vi "play_nPoint_id_slew_OL_FIFO.vi"() -> ()   [LabVIEW 2017]
uses:
  <vilib>/Analysis/Matrix/Datatypes/RealMatrix.ctl
  <vilib>/userdefined/High Color/nirio_resource_hc.ctl
  <vilib>/FPGAPlugInAG/cRIO-9082/niLvFpga_Open_cRIO-9082.vi
  <vilib>/rvi/interface/common/dynamic/niFpgaDynamicAddResources.vi
  <vilib>/FPGAPlugInAG/Dynamic/niLvFpga_Reset_Dynamic.vi
  <vilib>/rvi/interface/common/niFpgaWaitOnOcc.vi
  <vilib>/Utility/error.llb/Error Cluster From Error Code.vi
  <vilib>/rvi/errors/niLvFpgaAdjustHostInterfaceError.vi
  <vilib>/Analysis/Matrix/Numeric/Conversions/Matrix To Array - RM.vi
  <vilib>/FPGAPlugInAG/Dynamic/niLvFpga_Run_Dynamic.vi
  <vilib>/Analysis/Matrix/Numeric/Conversions/Array To Matrix - RA2.vi
  <vilib>/FPGAPlugInAG/Dynamic/niLvFpga_Close_Dynamic.vi
  <vilib>/rvi/interface/nirviOpenFPGA/nirviOpenFPGA.xnode
  FPGA Bitfiles/afmimagingcontro_FPGATargetSPARTA_IDOLFIFOinput_8nsqzYocPkw.lvbitx
  <vilib>/rvi/interface/nirviMethod/nirviMethod.xnode
  <vilib>/rvi/interface/nirviReadWriteControl/nirviReadWriteControl.xnode
  <vilib>/rvi/interface/nirviCloseFPGA/nirviCloseFPGA.xnode
  <vilib>/rvi/errors/niLvFpgaMergeErrorWithErrorCode.vi
  <vilib>/FPGAPlugInAG/Dynamic/niLvFpga_ConfigureFifo_Dynamic.vi
  <vilib>/rvi/interface/Simulation/niFpgaSimulationCallBeginRW.vi
  <vilib>/FPGAPlugInAG/Dynamic/niLvFpga_WriteFifo_Dynamic.vi
  <vilib>/FPGAPlugInAG/Dynamic/niLvFpga_ReadFifo_Dynamic.vi
  NiFpgaLv.dll
  <vilib>/Utility/file.llb/Read Delimited Spreadsheet (DBL).vi
  <vilib>/Analysis/Matrix/NI_Matrix.lvlib
  <vilib>/Utility/file.llb/Write Delimited Spreadsheet (DBL).vi
panel:
  out "stage_data_out":T1
  in  "u_in":T1
  in  "DAC-select":i16
  out "Timed Out?":bool
  out "Waveform Graph":dbl[](graph)
  out "Actual Depth 2":u32
  out "unsigned 16bit integer":u16
  out "Elements Remaining":u32
  out "Actual Depth":u32
  out "error out":errorcluster
  out "size(s) 3":i32[](array[numeric])
  out "x+y":i32
  out "YK TO":bool
  out "Unstable Traj":bool
  in  "traj_in_path":path
  out "AI1":T2(graph)
  out "size(s) 2":i32[](array[numeric])
  in  "data_out_path":path
  out "AI0":T2(graph)
  out "Waveform Chart":T2(graph)
  out "Loop Done":bool
  in  "Abort":bool
  in  "TsTicks":u32=1600
  out "y iter":i32
  out "size(s)":i32
  in  "umax":dbl=4.0 format="%#_13g"
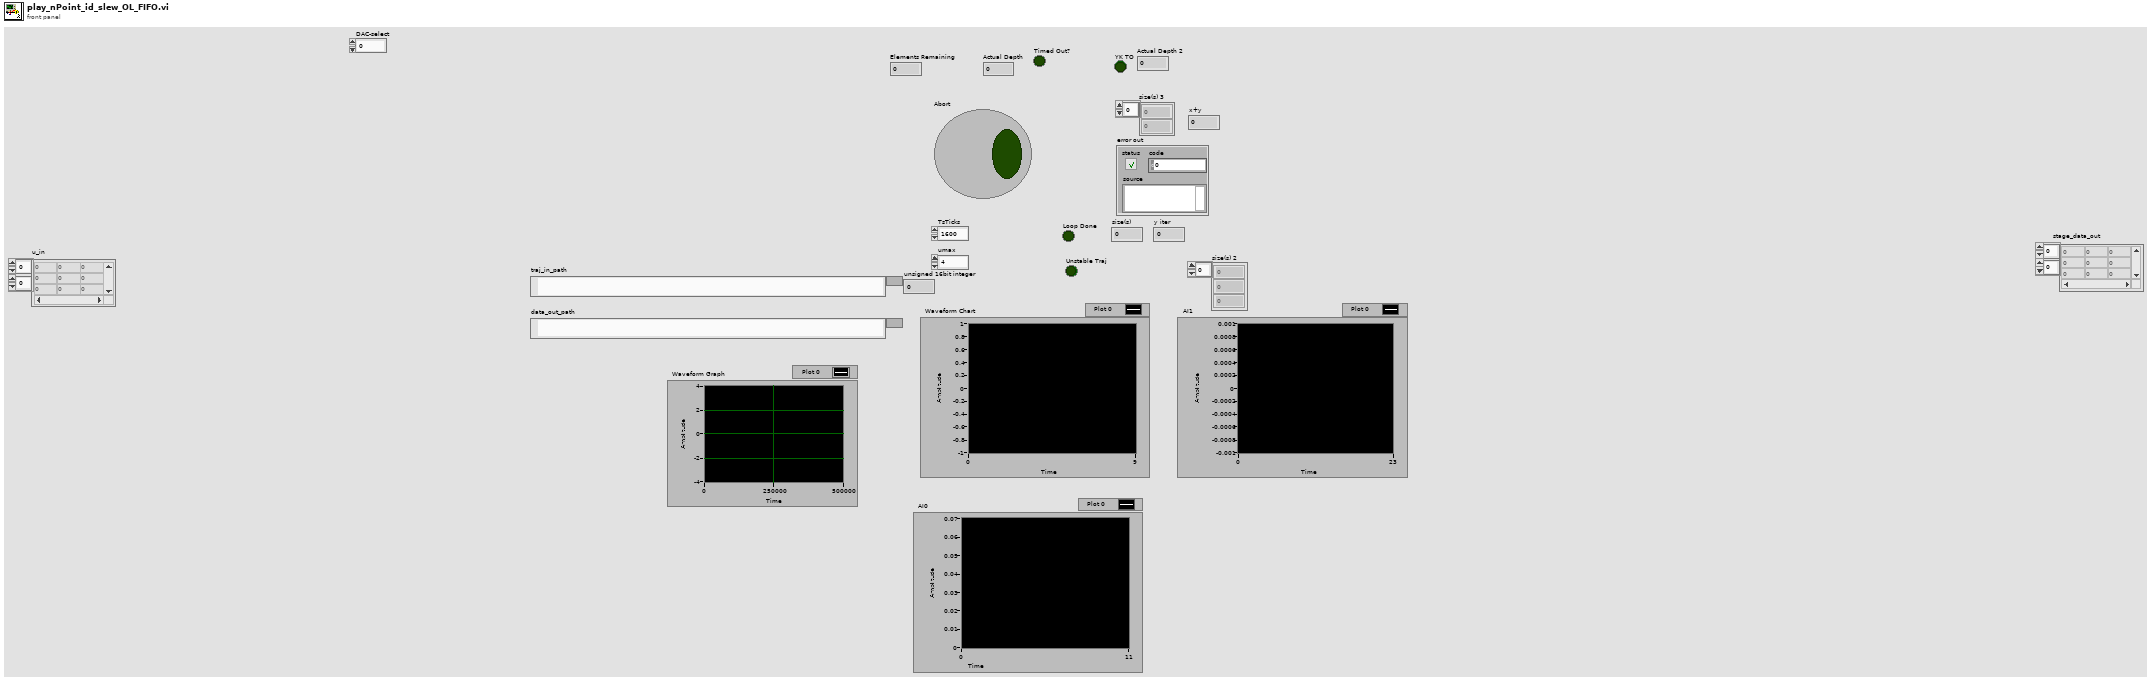
[diagram p1: front panel]
types:
  T1 = typedef "NI_Matrix.lvlib/RealMatrix.ctl" = dbl[][]
  T2 = cluster{"2D Data Out[0]":dbl, "2D Data Out[1]":dbl, "2D Data Out[2]":dbl, "2D Data Out[3]":dbl, "2D Data Out[4]":dbl, "2D Data Out[5]":dbl, "2D Data Out[6]":dbl, "2D Data Out[7]":dbl, "2D Data Out[8]":dbl}
  T3 = typedef "nirio_resource_hc.ctl" = tag
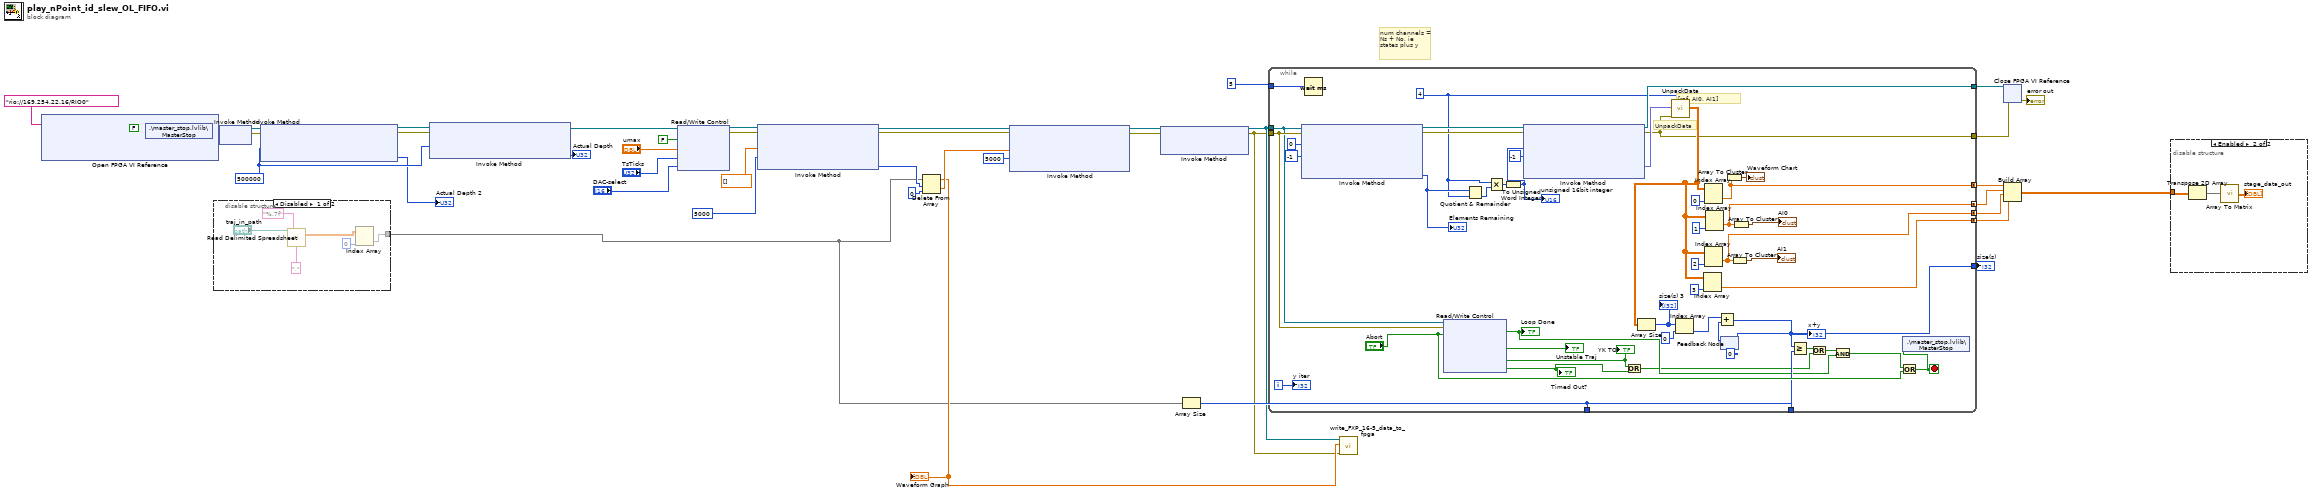
[diagram p0: block diagram]
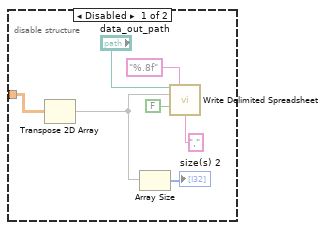
[diagram p2: hidden frame]
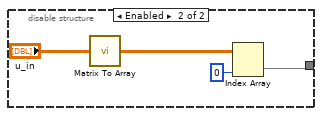
[diagram p3: hidden frame]
diagram:
  w29 = 500000
  # "num channels = Ns + No, ie states plus y"
  n1 = xnode "Open FPGA VI Reference"("resource name"=T3 "rio://169.254.22.16/RIO0") -> ("FPGA VI Reference Out"=w40:refnum<k20>, "error out"=w8:errorcluster)  [unwired: 1 in]
  n2 = shared-variable ".\\master_stop.lvlib\\MasterStop"(FALSE ("MasterStop"), error in=w8) -> (error out=w7:errorcluster)
  n3 = disable-structure shown="Disabled" {
    disable-tunnel: [w46 w51] -> w2
    frame Disabled {
      n4 = call-poly <vilib>:"Read Delimited Spreadsheet.vi"("file path (dialog if empty)"="traj_in_path", "format (%.3f)"="%.7f", "delimiter (\\t)"="," ("delimiter (\\t)")) -> ("all rows"=w45:dbl[][])  [unwired: 7 in, 5 out]
      n5 = Index Array(array=w45, index (col)=0 ("disabled index (col)")) -> (element=w46:dbl[])  [unwired: 1 in]
    }
    frame Enabled {
      n6 = call-poly <vilib>:"Matrix To Array.vi"("Real Matrix"="u_in") -> ("Real 2D Array"=w52:dbl[][])
      n7 = Index Array(array=w52, index (col)=0 ("disabled index (col)")) -> (element=w51:dbl[])  [unwired: 1 in]
    }
  }
  n8 = xnode "Invoke Method"("FPGA VI Reference In"=w40, "error in"=w7) -> ("FPGA VI Reference Out"=w38:refnum<k20>, "error out"=w37:errorcluster)
  n9 = xnode "Invoke Method"("FPGA VI Reference In"=w38, "error in"=w37, "Requested Depth"=w29) -> ("FPGA VI Reference Out"=w31:refnum<k20>, "error out"=w30:errorcluster, "Actual Depth"=→"Actual Depth 2":u32)
  n10 = xnode "Invoke Method"("FPGA VI Reference In"=w31, "error in"=w30, "Requested Depth"=w29) -> ("FPGA VI Reference Out"=w23:refnum<k20>, "Actual Depth"=→"Actual Depth":u32)  [unwired: 1 out]
  n11 = xnode "Read/Write Control"("FPGA VI Reference In"=w23, "Abort"=FALSE, "ymax"="umax", "TsTicks"="TsTicks", "DAC-select"="DAC-select") -> ("FPGA VI Reference Out"=w22:refnum<k20>, "error out"=w21:errorcluster)  [unwired: 1 in]
  n12 = xnode "Invoke Method"("FPGA VI Reference In"=w22, "error in"=w21, "Data"=sgl[] [], "Timeout (ms)"=5000) -> ("FPGA VI Reference Out"=w18:refnum<k20>, "error out"=w17:errorcluster, "Empty Elements Remaining"=w12:u32)
  n13 = Delete From Array(array=w2, length=w12, index=0) -> (deleted portion=w13:dbl[], array with subset deleted=w4:dbl[])
  "Waveform Graph" <- w4
  n14 = xnode "Invoke Method"("FPGA VI Reference In"=w18, "error in"=w17, "Data"=w13, "Timeout (ms)"=5000) -> ("FPGA VI Reference Out"=w16:refnum<k20>, "error out"=w15:errorcluster)  [unwired: 1 out]
  n15 = xnode "Invoke Method"("FPGA VI Reference In"=w16, "error in"=w15) -> ("FPGA VI Reference Out"=w5:refnum<k20>, "error out"=w3:errorcluster)  [unwired: 1 in]
  n16 = Array Size(array=w2) -> (size(s)=w27:i32)
  n17 = while {
    tunnel: 5 -> [w100]
    tunnel: w5 -> [w80]
    tunnel: w3 -> [w81]
    tunnel: [w60] -> w35
    tunnel: [w92] -> w42
    tunnel: [w66] -> w41
    tunnel: [w74] -> w34 mode=concatenating
    tunnel: [w73] -> w33 mode=concatenating
    tunnel: [w70] -> w32 mode=concatenating
    tunnel: [w67] -> w28 mode=concatenating
    tunnel: w27 -> [_]
    tunnel: w27 -> [w65]
    i -> [w83]
    stop <- w58 stop-if-true
    w82 = u32 4 ("y")
    # "[ref, AI0, AI1]"
    # "UnpackData"
    n18 = xnode "Invoke Method"("FPGA VI Reference In"=w80, "error in"=w81, "Number of Elements"=0 ("Timeout (ms)"), "Timeout (ms)"=-1) -> ("FPGA VI Reference Out"=w96:refnum<k20>, "error out"=w97:errorcluster, "Elements Remaining"=w89:u32)  [unwired: 1 out]
    "Elements Remaining" <- w89
    n19 = Wait (ms)(milliseconds to wait=w100) -> ()  [unwired: 1 out]
    n20 = xnode "Read/Write Control"("FPGA VI Reference In"=w80, "error in"=w81, "Abort"="Abort") -> ("Loop Done"=w59:bool, "Unstable Traj"=→"Unstable Traj":bool, "YK TO"=w57:bool, "Timed Out?"=w55:bool)  [unwired: 2 out]
    "Loop Done" <- w59
    "YK TO" <- w57
    "Timed Out?" <- w55
    n21 = Quotient & Remainder(x=w89, y=w82) -> (floor(x/y)=w90:u32)  [unwired: 1 out]
    n22 = Multiply(x=w82, y=w90) -> (x*y=w94:u32)
    n23 = To Unsigned Word Integer(number=w94) -> (unsigned 16bit integer=w91:u16)
    "unsigned 16bit integer" <- w91
    n24 = xnode "Invoke Method"("FPGA VI Reference In"=w96, "error in"=w97, "Number of Elements"=w91, "Timeout (ms)"=-1) -> ("FPGA VI Reference Out"=w92:refnum<k20>, "error out"=w60:errorcluster, "Data"=w88:fxp<+/-,16,5>[])  [unwired: 1 out]
    n25 = Or(x=w57, y=w55) -> (x .or. y?=w56:bool)
    n26 = call "UnpackData.vi"("NumChannels"=w82, "error In"=w60, "1D Data In"=w88) -> ("2D Data Out"=w68:dbl[][])  [unwired: 7 in, 1 out]
    n27 = Array Size(array=w68) -> (size(s)=w87:i32[])
    "size(s) 3" <- w87
    n28 = Index Array(array=w87, index=0) -> (element=w85:i32)
    n29 = Index Array(array=w68, index (col)=3 ("disabled index (col)")) -> (element=w67:dbl[])  [unwired: 1 in]
    n30 = Index Array(array=w68, index (col)=2 ("disabled index (col)")) -> (element=w70:dbl[])  [unwired: 1 in]
    n31 = Index Array(array=w68, index (col)=0 ("disabled index (col)")) -> (element=w74:dbl[])  [unwired: 1 in]
    n32 = Index Array(array=w68, index (col)=1 ("disabled index (col)")) -> (element=w73:dbl[])  [unwired: 1 in]
    n33 = feedback #1(0) -> (w86:i32)
    n34 = Add(x=w85, y=w86) -> (x+y=w66:i32)
    "x+y" <- w66
    n35 = feedback-in #1(w66) -> ()
    n36 = Array To Cluster(array=w74) -> (cluster=→"Waveform Chart":T2)
    n37 = Array To Cluster(array=w70) -> (cluster=→"AI1":T2)
    n38 = Array To Cluster(array=w73) -> (cluster=→"AI0":T2)
    n39 = Greater Or Equal?(x=w66, y=w65) -> (x >= y?=w64:bool)
    n40 = Or(x=w64, y=w56) -> (x .or. y?=w62:bool)
    n41 = And(x=w62, y=w59) -> (x .and. y?=w61:bool)
    n42 = Or(x=w61, y="Abort") -> (x .or. y?=w58:bool)
    n43 = shared-variable ".\\master_stop.lvlib\\MasterStop"(w58) -> ()  [unwired: 1 in, 1 out]
    "y iter" <- w83
  }
  "size(s)" <- w41
  n44 = call "write_FXP_16-5_data_to_fpga.vi"("error in"=w3, "all rows"=w4, "FPGA Interface"=w5) -> ()  [unwired: 7 in, 2 out]
  n45 = xnode "Close FPGA VI Reference"("FPGA VI Reference In"=w42, "error in"=w35) -> ("error out"=→"error out":errorcluster)
  n46 = Build Array(w34, w33, w32, w28) -> (w1:dbl[][])
  n47 = disable-structure shown="Enabled" {
    disable-tunnel: w1 -> [w102 w108]
    frame Disabled {
      n48 = Transpose 2D Array(2D array=w102) -> (transposed array=w101:dbl[][])
      n49 = Array Size(array=w101) -> (size(s)=→"size(s) 2":i32[])
      n50 = call-poly <vilib>:"Write Delimited Spreadsheet.vi"("file path (dialog if empty)"="data_out_path", "format (%.3f)"="%.8f", "2D data"=w101, "append to file? (new file:F)"=FALSE, "delimiter (\\t)"="," ("delimiter (\\t)")) -> ()  [unwired: 9 in, 2 out]
    }
    frame Enabled {
      n51 = Transpose 2D Array(2D array=w108) -> (transposed array=w109:dbl[][])
      n52 = call-poly <vilib>:"Array To Matrix.vi"("Real 2D Array"=w109) -> ("Real Matrix"=→"stage_data_out":T1)
    }
  }
